vi "Interframe_template-matched-tempbox_displacements_FTMethod_Checked_VI.vi"() -> ()   [LabVIEW 2012]
uses:
  <vilib>/Utility/file.llb/Write To Spreadsheet File (I64).vi
  <vilib>/imath/engines/lvmath2/RunTimeEngine/NodeEndStatement/NIMS_NodeEndStatement_Output.vi
  <instcachedir>/0/NIMS_NodeEndStatement_Output_53EC0D466D134D7ABD903AC30B43404B.lvgen/NIMS_NodeEndStatement_Output_53EC0D466D134D7ABD903AC30B43404B_004.vi
  <vilib>/imath/engines/lvmath2/RunTimeEngine/ErrorHandling/NIMS_Finalize Error.vi
  <vilib>/imath/engines/lvmath2/RunTimeEngine/ArithmeticOperatorToken/NIMS_ArithmeticOperator_minus.vi
  <instcachedir>/0/NIMS_ArithmeticOperator_minus_E353D3D62E0E432C853B0E64BA14CDF8.lvgen/NIMS_ArithmeticOperator_minus_E353D3D62E0E432C853B0E64BA14CDF8_007.vi
  <vilib>/imathl/engines/lvmath/Functions/Error Handling/Create Error.vi
  <instcachedir>/0/NIMS_NodeEndStatement_Output_53EC0D466D134D7ABD903AC30B43404B.lvgen/NIMS_NodeEndStatement_Output_53EC0D466D134D7ABD903AC30B43404B_002.vi
panel:
  out "RAY":dbl[][](array[numeric])
  out "Frame\nDelta_X\nDelta_Z":i16[][](array[numeric])
  out "Matched TempBox (z,x): ROI-Frame_of_Reference":u8[][](array[numeric])
  out "Max_RAY":dbl[](array[numeric])
  out "Delta_Z (TempBox-Template)":i16[](array[numeric])
  out "Delta_X (TempBox-Template)":i16[](array[numeric])
  out "RAY_1Darray":dbl[](array[numeric])
  in  "ROI in\n2nd frame\n    e_z":u16=301
  in  "ROI in\n2nd frame\n    s_z":u16=272
  in  "ROI in\n2nd frame\n    e_x":u16=727
  in  "ROI in\n2nd frame\n    s_x":u16=623
  in  "?":bool
  in  "1st frame":u16=153
  in  "Last frame":u16=154
  out "Frames":T1(plugin-control)
  out "Template in 1st frame of every iteration":u8[][](array[numeric])
  in  "Template \n      in\n1st frame\n     s_x":u16=658
  in  "Template \n      in \n1st frame\n    s_z":u16=282
  in  "Template \n      in \n1st frame\n    e_x":u16=692
  in  "Template \n      in \n1st frame\n    e_z":u16=291
  out "framesPerSecond":u16
  out "Image Type":T2 items=["Grayscale (U8)", "Grayscale (I16)", "Grayscale (SGL)", "Complex (CSG)", "RGB (U32)", "HSL (U32)", "RGB (U64)"]
  out "Number of Frames":u16
  in  "Path":path=path "C:/Users/admin/Desktop/lohit/pat3.avi"
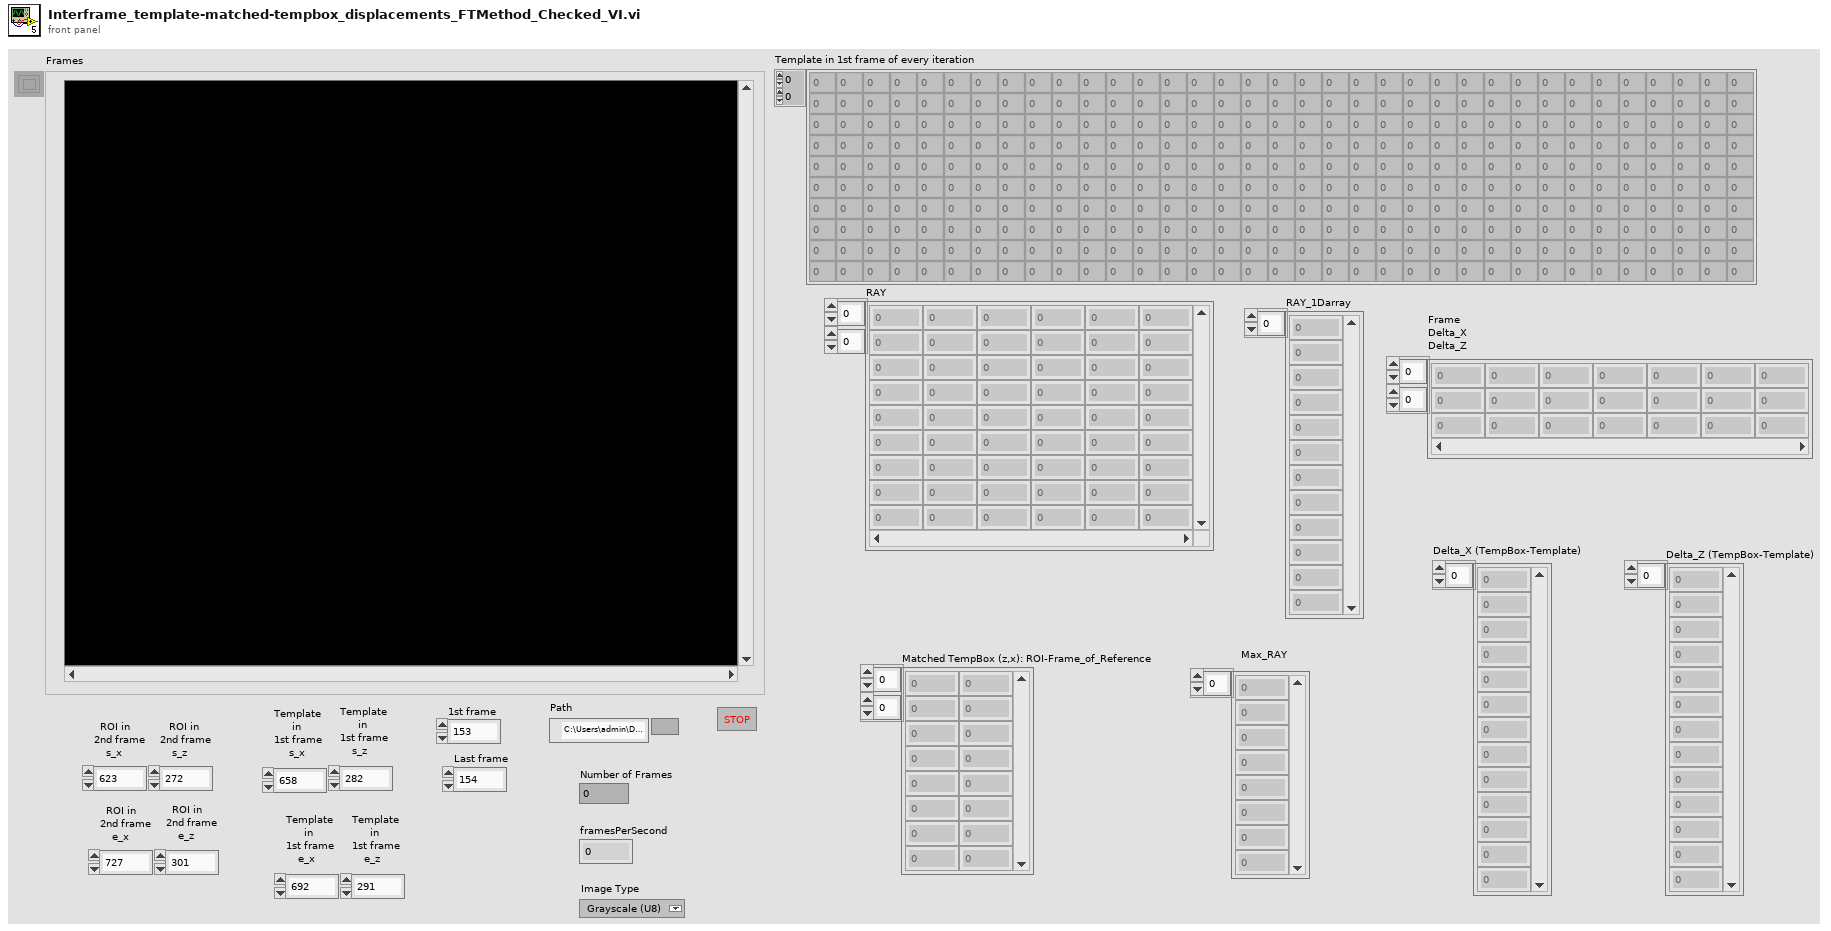
[diagram p1: front panel]
types:
  T1 = typedef "IMAQ Image.ctl" = refnum<image>
  T2 = typedef "Image Type" = u32
  T3 = typedef "AviRefnum.ctl" = refnum<k1>
  T4 = cluster{"width":u32, "height":u32, "framesPerSecond":u32, "compressionFilter":string, "hasData":bool}
  T5 = cluster{"[0]":i32, "[1]":i32, "[2]":i32, "[3]":i32, "[4]":i32, "[5]":i32, "[6]":i32, "[7]":i32, "[8]":i32}
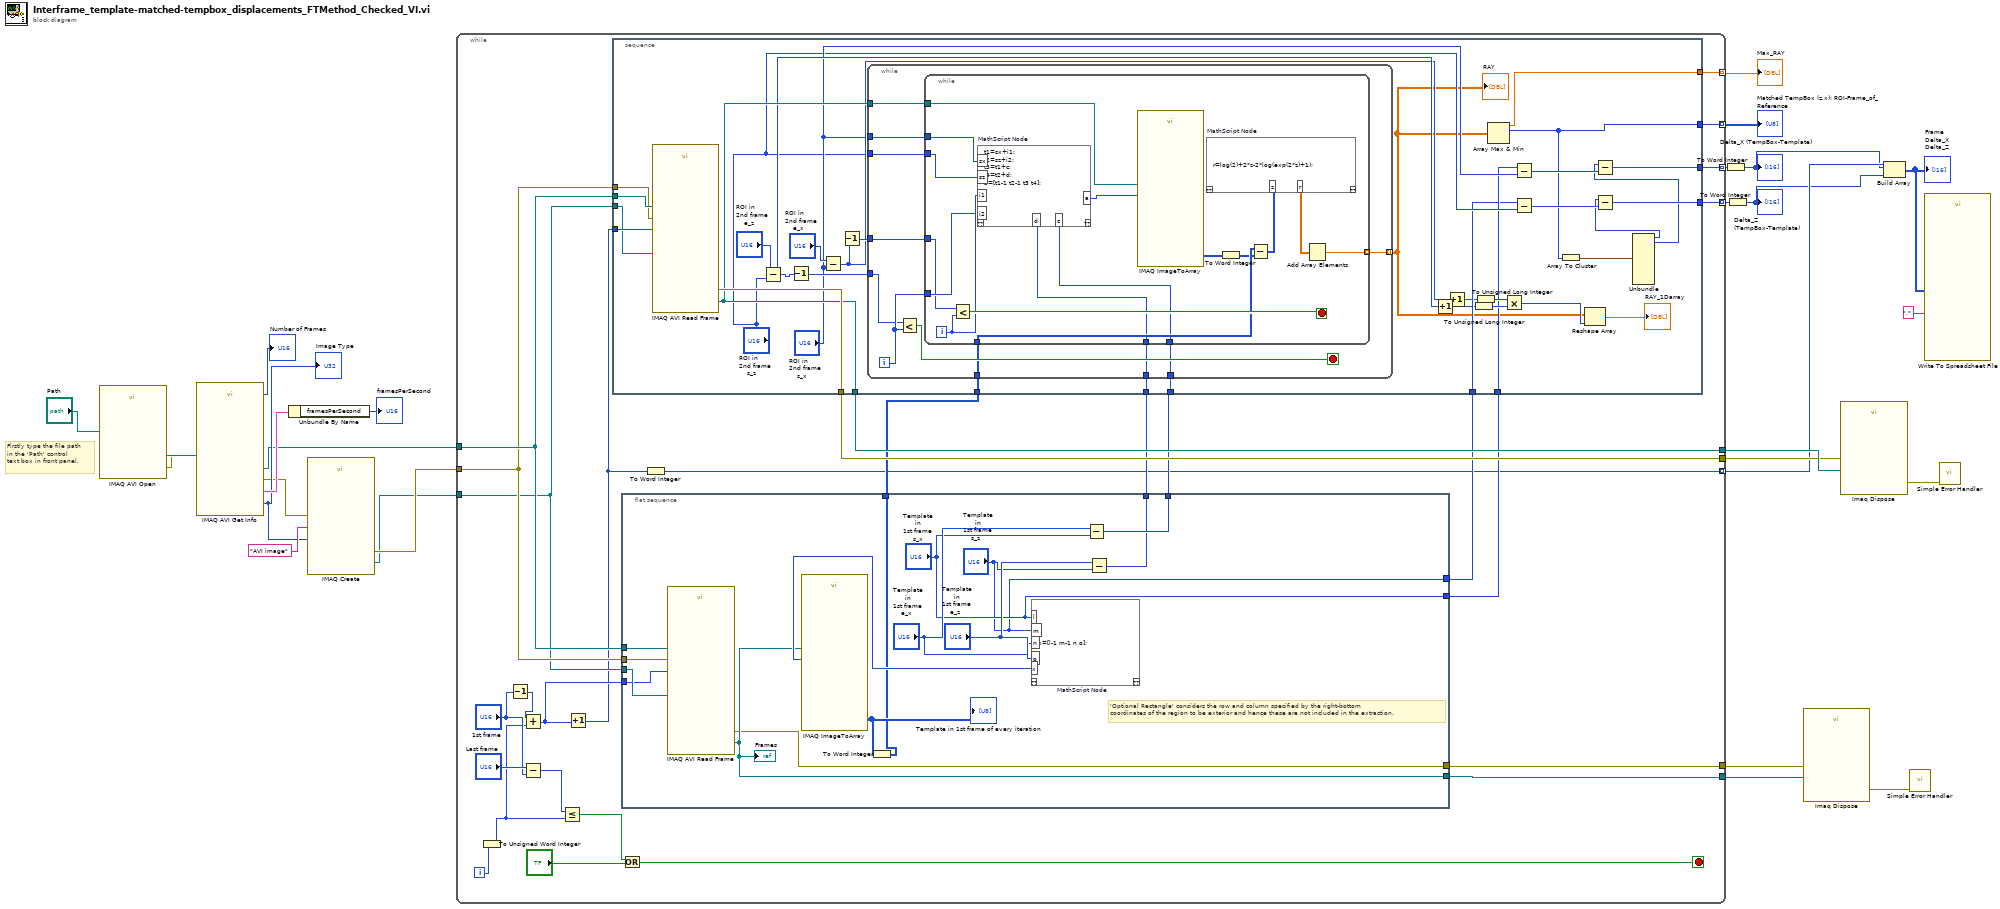
[diagram p0: block diagram]
diagram:
  # "Firstly type the file path\nin the 'Path' control \ntext box in front panel."
  n1 = call "IMAQ AVI Open"("AVI Path"="Path") -> ("error out"=w20:errorcluster, "Avi Refnum"=w26:T3)  [unwired: 9 in]
  n2 = call "IMAQ AVI Get Info"("error in (no error)"=w20, "Avi Refnum"=w26) -> ("error out"=w19:errorcluster, "Image Type"=w22:T2, "Number of Frames"=→"Number of Frames":u32, "Avi Refnum (duplicate)"=w18:T3, "Frame Data"=w24:T4)  [unwired: 5 in]
  "Image Type" <- w22
  n3 = Unbundle By Name(w24) -> ("framesPerSecond"=→"framesPerSecond":u32)
  n4 = call "IMAQ Create"("Image Name"="AVI image", "Image Type"=w22, "error in (no error)"=w19) -> ("New Image"=w16:T1, "error out"=w17:errorcluster)  [unwired: 2 in]
  n5 = while {
    tunnel: w18 -> [w43]
    tunnel: w17 -> [w42]
    tunnel: w16 -> [w41]
    tunnel: [w54] -> w14
    tunnel: [w53] -> w13
    tunnel: [w52] -> w10 mode=indexing
    tunnel: [w51] -> w9 mode=indexing
    tunnel: [w30] -> w11 mode=indexing
    tunnel: [w38] -> w8
    tunnel: [w37] -> w7
    tunnel: [w29] -> w4 mode=indexing
    tunnel: [w28] -> w3 mode=indexing
    i -> [w46]
    stop <- w55 stop-if-true
    n6 = To Unsigned Word Integer(number=w46) -> (unsigned 16bit integer=w31:u16)
    n7 = Decrement(x="1st frame") -> (x-1=w48:u16)
    n8 = Add(x=w48, y=w31) -> (x+y=w40:u16)
    n9 = Subtract(x="Last frame", y="1st frame") -> (x-y=w49:u16)
    n10 = Less Or Equal?(x=w49, y=w31) -> (x <= y?=w44:bool)
    n11 = Increment(x=w40) -> (x+1=w39:u16)
    n12 = stacked-sequence {
      tunnel: w43 -> [w135]
      tunnel: w42 -> [w133]
      tunnel: w41 -> [w134]
      tunnel: w39 -> [w136]
      tunnel: [w131] -> w54
      tunnel: [w132] -> w53
      tunnel: [w129] -> w52
      tunnel: [w128] -> w51
      tunnel: w36 -> [w114]
      tunnel: w33 -> [w113]
      tunnel: w32 -> [w112]
      tunnel: w35 -> [w111]
      tunnel: w34 -> [w110]
      tunnel: [w106] -> w29
      tunnel: [w105] -> w28
      frame #0 {
        n13 = call "IMAQ AVI Read Frame"("error in (no error)"=w133, "Frame Number"=w136, "Image"=w134, "Avi Refnum"=w135) -> ("error out"=w132:errorcluster, "Image Out"=w131:T1)  [unwired: 4 in, 2 out]
        n14 = Subtract(x="ROI in\n2nd frame\n    e_z", y="ROI in\n2nd frame\n    s_z") -> (x-y=w122:u16)
        n15 = Decrement(x=w122) -> (x-1=w123:u16)
        n16 = Subtract(x="ROI in\n2nd frame\n    e_x", y="ROI in\n2nd frame\n    s_x") -> (x-y=w119:u16)
        n17 = Decrement(x=w119) -> (x-1=w120:u16)
        n18 = while {
          tunnel: w131 -> [w146]
          tunnel: w114 -> [w144]
          tunnel: w111 -> [w143]
          tunnel: w110 -> [w142]
          tunnel: [w141] -> w107 mode=indexing
          tunnel: w123 -> [w140]
          tunnel: w120 -> [w139]
          tunnel: "ROI in\n2nd frame\n    s_x" -> [w138]
          tunnel: "ROI in\n2nd frame\n    s_z" -> [w137]
          i -> [w145]
          stop <- w147 stop-if-true
          n19 = Less?(x=w140, y=w145) -> (x < y?=w147:bool)
          n20 = while {
            tunnel: w146 -> [w161]
            tunnel: w145 -> [w159]
            tunnel: w144 -> [w157]
            tunnel: w143 -> [w155]
            tunnel: w142 -> [w154]
            tunnel: [w153] -> w141 mode=indexing
            tunnel: w139 -> [w152]
            tunnel: w138 -> [w151]
            tunnel: w137 -> [w150]
            i -> [w160]
            stop <- w162 stop-if-true
            n21 = Less?(x=w152, y=w160) -> (x < y?=w162:bool)
            n22 = mathscript code="t1=sx+i1;\nt2=sz+i2;\nt3=t1+c;\nt4=t2+d;\na=[t1-1 t2-1 t3 t4];"("sx"=w151, "sz"=w150, "i1"=w160, "i2"=w159, "c"=w155, "d"=w154) -> ("a"=w158:i32[])  [unwired: 1 in, 1 out]
            n23 = call "IMAQ ImageToArray"("Optional Rectangle"=w158, "Image"=w161) -> ("Image Pixels (U8)"=w163:u8[][])  [unwired: 2 in, 4 out]
            n24 = To Word Integer(number=w163) -> (16bit integer=w156:i16[][])
            n25 = Subtract(x=w157, y=w156) -> (x-y=w149:i16[][])
            n26 = mathscript code="r=log(2)+2*z-2*log(exp(2*z)+1);"("z"=w149) -> ("r"=w148:dbl[][])  [unwired: 1 in, 1 out]
            n27 = Add Array Elements(numeric array=w148) -> (sum=w153:dbl)
          }
        }
        "RAY" <- w107
        n28 = Increment(x=w122) -> (x+1=w109:u16)
        n29 = Increment(x=w119) -> (x+1=w108:u16)
        n30 = To Unsigned Long Integer(number=w109) -> (unsigned 32bit integer=w125:u32)
        n31 = To Unsigned Long Integer(number=w108) -> (unsigned 32bit integer=w126:u32)
        n32 = Array Max & Min(array=w107) -> (max value=w106:dbl, max index (indices)=w105:i32[])  [unwired: 2 out]
        n33 = Multiply(x=w126, y=w125) -> (x*y=w127:u32)
        n34 = Subtract(x=w113, y="ROI in\n2nd frame\n    s_x") -> (x-y=w117:u16)
        n35 = Subtract(x=w112, y="ROI in\n2nd frame\n    s_z") -> (x-y=w118:u16)
        n36 = Array To Cluster(array=w105) -> (cluster=w130:T5)
        n37 = Reshape Array "Reshape Array"(w107, w127) -> (→"RAY_1Darray":dbl[])
        n38 = Unbundle "Unbundle"(w130) -> ("[0]"=w104:i32, "[1]"=w103:i32)  [unwired: 7 out]
        n39 = Subtract(x=w103, y=w117) -> (x-y=w129:i32)
        n40 = Subtract(x=w104, y=w118) -> (x-y=w128:i32)
      }
    }
    n41 = flat-sequence {
      tunnel: w43 -> [w67]
      tunnel: w42 -> [w66]
      tunnel: w41 -> [w65]
      tunnel: w40 -> [w64]
      tunnel: [w63] -> w38
      tunnel: [w62] -> w37
      tunnel: [w61] -> w36
      tunnel: [w59] -> w35
      tunnel: [w58] -> w34
      tunnel: ["Template \n      in\n1st frame\n     s_x"] -> w33
      tunnel: ["Template \n      in \n1st frame\n    s_z"] -> w32
      frame #0 {
        # "'Optional Rectangle' considers the row and column specified by the right-bottom\ncoordinates of the region to be exterior and hence these are not included in the extraction."
        n42 = call "IMAQ AVI Read Frame"("error in (no error)"=w66, "Frame Number"=w64, "Image"=w65, "Avi Refnum"=w67) -> ("error out"=w62:errorcluster, "Image Out"=w63:T1)  [unwired: 4 in, 2 out]
        "Frames" <- w63
        n43 = mathscript code="x=[l-1 m-1 n o];"("l"="Template \n      in\n1st frame\n     s_x", "m"="Template \n      in \n1st frame\n    s_z", "n"="Template \n      in \n1st frame\n    e_x", "o"="Template \n      in \n1st frame\n    e_z") -> ("x"=w69:i32[])  [unwired: 1 in, 1 out]
        n44 = call "IMAQ ImageToArray"("Optional Rectangle"=w69, "Image"=w63) -> ("Image Pixels (U8)"=w70:u8[][])  [unwired: 2 in, 4 out]
        "Template in 1st frame of every iteration" <- w70
        n45 = To Word Integer(number=w70) -> (16bit integer=w61:i16[][])
        n46 = Subtract(x="Template \n      in \n1st frame\n    e_x", y="Template \n      in\n1st frame\n     s_x") -> (x-y=w59:u16)
        n47 = Subtract(x="Template \n      in \n1st frame\n    e_z", y="Template \n      in \n1st frame\n    s_z") -> (x-y=w58:u16)
      }
    }
    n48 = Or(x=w44, y="?") -> (x .or. y?=w55:bool)
    n49 = To Word Integer(number=w39) -> (16bit integer=w30:i16)
  }
  "Max_RAY" <- w4
  "Matched TempBox (z,x): ROI-Frame_of_Reference" <- w3
  n50 = To Word Integer(number=w10) -> (16bit integer=w5:i16[])
  "Delta_X (TempBox-Template)" <- w5
  n51 = To Word Integer(number=w9) -> (16bit integer=w6:i16[])
  "Delta_Z (TempBox-Template)" <- w6
  n52 = call "Imaq Dispose"("Image"=w8, "error in (no error)"=w7) -> ("error out"=w12:errorcluster)  [unwired: 4 in]
  n53 = call "Imaq Dispose"("Image"=w14, "error in (no error)"=w13) -> ("error out"=w15:errorcluster)  [unwired: 4 in]
  n54 = Build Array "Build Array"(w11, w5, w6) -> (w1:i16[][])
  "Frame\nDelta_X\nDelta_Z" <- w1
  n55 = call <vilib>:"Simple Error Handler.vi"("error in (no error)"=w12) -> ()  [unwired: 4 in, 5 out]
  n56 = call-poly <vilib>:"Write To Spreadsheet File.vi"("delimiter (\\t)"="," ("delimiter (\\t)"), "2D data"=w1) -> ()  [unwired: 6 in, 1 out]
  n57 = call <vilib>:"Simple Error Handler.vi"("error in (no error)"=w15) -> ()  [unwired: 4 in, 5 out]
